vi "质控数据起始时间戳查询.vi"() -> (0 "加标回收索引起始时间":string, 1 "标样核查索引起始时间":string, 2 "零点核查索引起始时间":string, 3 "跨度核查索引起始时间":string)   [LabVIEW 2016, in "数据传输系统-04.lvlib"]
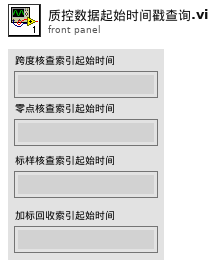
[diagram p1: front panel]
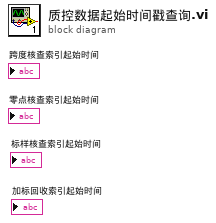
[diagram p0: block diagram]
diagram:
